vi "OAT Order Power Spectrum (N Channels).vi"(0 "even-angle signals":cluster{"r0":dbl, "dr":dbl, "Y":dbl[]}[](array[cluster]) {"r0" format="%.2p"; "dr" format="%.2p"; "Y" format="%.2f"}, 1 "dB on? (T)":bool=TRUE, 5 "even-angle channel info":T8[](array[typedef]) {"channel info"."pregain" format="%.2f"; "channel info"."weighting filter" items=["Linear", "A-weighting", "B-weighting", "C-weighting", "ITU-R 468-4", "Dolby", "CCITT", "C-message", "Wb", "Wc", "Wd", "We", "Wf", "Wh", "Wj", "Wk", "Wm", "AES17 20 kHz lowpass", "AES17 40 kHz lowpass", "AES17 20 kHz highpass", "AES17 40 kHz highpass"]; "channel info"."dB reference" format="%^.1e"; "channel info"."engineering units" items=["custom..."=0, "V"=1, "A"=21, "C"=30, "pC"=31, "s"=32, "-"=29, "Pa"=2, "N"=20, "g"=3, "m/s^2"=4, "m/s"=5, "m"=6, "mm/s"=12, "mm"=13, "micron/s"=14, "micron"=15, "in/s^2"=7, "in/s"=8, "in"=9, "mil/s"=10, "mil"=11, "rad/s^2"=16, "rad/s"=17, "rad"=18, "deg/s^2"=26, "deg/s"=27, "deg"=28, "RPM"=22, "cycle/s^2"=23, "Hz"=24, "cycle"=25, "strain"=19]; "channel info"."sensor sensitivity" format="%#_5f"}, 7 "window":u32(ring)=1 items=["None"=0, "Hanning"=1, "Hamming"=2, "Blackman-Harris"=3, "Exact Blackman"=4, "Blackman"=5, "Flat Top"=6, "4 Term B-Harris"=7, "7 Term B-Harris"=8, "Low Sidelobe"=9, "Gaussian"=62], 9 "block size":i32=1024 min=2, 11 "error in (no error)":errorcluster, 12 "averaging parameters":T7={"averaging mode"=enum."No averaging", "weighting mode"=enum."Exponential", "number of averages"=10, "linear mode"=enum."One shot"} {"number of averages" min=1 step=1}, 13 "restart averaging? (F)":bool) -> (3 "new spectrum available?":bool, 4 "order power spectra":T10(array[cluster]) {"order 0" format="%.2p"; "delta order" format="%.2p"; "magnitude" format="%.2f"}, 6 "unit labels":string[](array[string]), 8 "averages completed":dbl, 10 "spectrum info":T1[](array[typedef]) {"x-axis units" items=["Time (s)"=0, "Frequency-CB (Hz)"=1, "Frequency-CPB (Hz)"=1248, "Frequency-Arbitrary (Hz)"=2357, "Quefrency (s)"=2, "Revolutions (rev)"=3, "Order"=4, "Speed (RPM)"=11, "Speed (rad/s)"=21, "Index"=65535]; "weighting filter" items=["Linear", "A-weighting", "B-weighting", "C-weighting", "ITU-R 468-4", "Dolby", "CCITT", "C-message", "Wb", "Wc", "Wd", "We", "Wf", "Wh", "Wj", "Wk", "Wm", "AES17 20 kHz lowpass", "AES17 40 kHz lowpass", "AES17 20 kHz highpass", "AES17 40 kHz highpass"]; "dB reference [EU]" format="%.2f"; "engineering units" items=["custom..."=0, "V"=1, "A"=21, "C"=30, "pC"=31, "s"=32, "-"=29, "Pa"=2, "N"=20, "g"=3, "m/s^2"=4, "m/s"=5, "m"=6, "mm/s"=12, "mm"=13, "micron/s"=14, "micron"=15, "in/s^2"=7, "in/s"=8, "in"=9, "mil/s"=10, "mil"=11, "rad/s^2"=16, "rad/s"=17, "rad"=18, "deg/s^2"=26, "deg/s"=27, "deg"=28, "RPM"=22, "cycle/s^2"=23, "Hz"=24, "cycle"=25, "strain"=19]; "spectral info"."window" items=["None "=0, "Hanning"=1, "Hamming"=2, "Blackman-Harris"=3, "Exact Blackman"=4, "Blackman"=5, "Flat Top"=6, "4 Term B-Harris "=7, "7 Term B-Harris"=8, "Low Sidelobe"=9, "Force - Exponential"=10, "Gaussian"=62]}, 14 "averaging done?":bool, 15 "error out":errorcluster)   [LabVIEW 2017, in "SoundVib_OrderTracking.lvlib"]
doc: "Computes the order power spectrum of an even-angle signal. Wire data to the <B>even-angle signal</B> input to determine the polymorphic instance to use or manually select the instance."
uses:
  <vilib>/addons/Sound and Vibration/Order Analysis/Resample Order Tracking/SoundVib_OrderTracking.lvlib
  <vilib>/addons/_NISVFA/_Shared subVIs/Controls/svc_Resampled Channel Info.ctl
  <vilib>/addons/_NISVFA/_Shared subVIs/Controls/svc_Channel Info.ctl
  <vilib>/addons/_NISVFA/_Shared subVIs/Controls/svc_Engineering Units Text Ring.ctl
  <vilib>/addons/_NISVFA/_Shared subVIs/Controls/svc_Weighting Filter Text Ring.ctl
  <vilib>/addons/_NISVFA/_Shared subVIs/Controls/svc_Spectrum Info.ctl
  <vilib>/addons/_NISVFA/_Shared subVIs/Controls/svc_X-Axis Units.ctl
  <vilib>/addons/_NISVFA/_Shared subVIs/Controls/svc_Spectrum Type.ctl
  <vilib>/addons/_NISVFA/_Shared subVIs/Controls/svc_Complimentary Spectrum Units.ctl
  <vilib>/addons/Sound and Vibration/Order Analysis/Resample Order Tracking/SoundVib_Resampling.lvlib
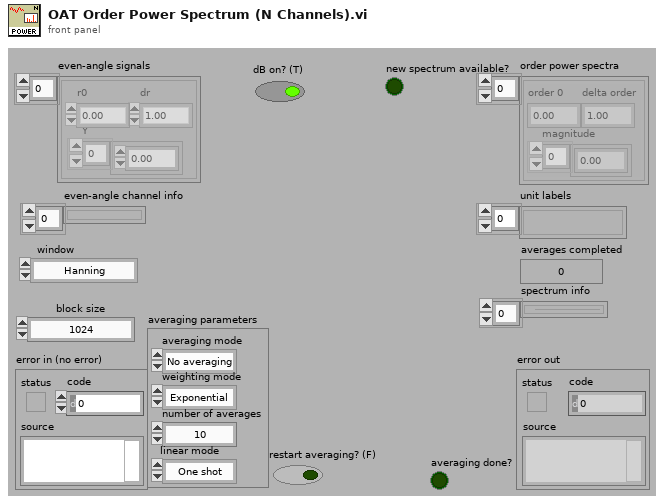
[diagram p1: front panel]
types:
  T1 = typedef "svc_Spectrum Info.ctl" = cluster{"channel name":string, "description":string, "x-axis units":T2, "spectral info":cluster{"spectrum type":T3, "linear/dB":enum16{"linear", "dB"}, "window":u16, "window size":i32, "FFT size":i32}, "engineering units":T4, "custom label":string, "dB reference [EU]":dbl, "peak units":enum16{"rms", "peak", "peak-peak"}, "weighting filter":T5, "spectral density?":bool, "unit label":string, "spectrum skewed?":bool, "complimentary spectrum units":T6}
  T2 = typedef "svc_X-Axis Units.ctl" = u16
  T3 = typedef "svc_Spectrum Type.ctl" = enum16{"FFT Spectrum [complex]", "Amplitude [Magnitude]", "Power [Magnitude^2]", "Cross Spectrum [complex]", "Frequency Response [Complex]"}
  T4 = typedef "svc_Engineering Units Text Ring.ctl" = u16
  T5 = typedef "svc_Weighting Filter Text Ring.ctl" = u16
  T6 = typedef "svc_Complimentary Spectrum Units.ctl" = enum16{"none", "radians", "degrees", "cycles", "imaginary"}
  T7 = cluster{"averaging mode":enum16{"No averaging", "Vector averaging", "RMS averaging", "Peak hold"}, "weighting mode":enum16{"Linear", "Exponential"}, "number of averages":u32, "linear mode":enum16{"One shot", "Auto restart"}}
  T8 = typedef "svc_Resampled Channel Info.ctl" = cluster{"channel name":string, "description":string, " channel info":T9}
  T9 = typedef "svc_Channel Info.ctl" = cluster{"sensor sensitivity":dbl, "engineering units":T4, "dB reference":dbl, "custom label":string, "weighting filter":T5, "pregain":dbl}
  T10 = cluster{"order 0":dbl, "delta order":dbl, "magnitude":dbl[]}[]
  T11 = cluster{"ignore dt":bool, "ignore t0 continuity":bool, "ignore array length":bool, "ignore channel info":bool, "ignore channel name":bool}
  T12 = cluster{"ignore dt's equal":bool, "ignore array lengths equal":bool, "ignore # channels":bool}
  T13 = cluster{"r0":dbl, "dr":dbl, "even angle signal":dbl[]}[]
  T14 = enum16{"Restart processing", "Continue processing", "Skip processing"}
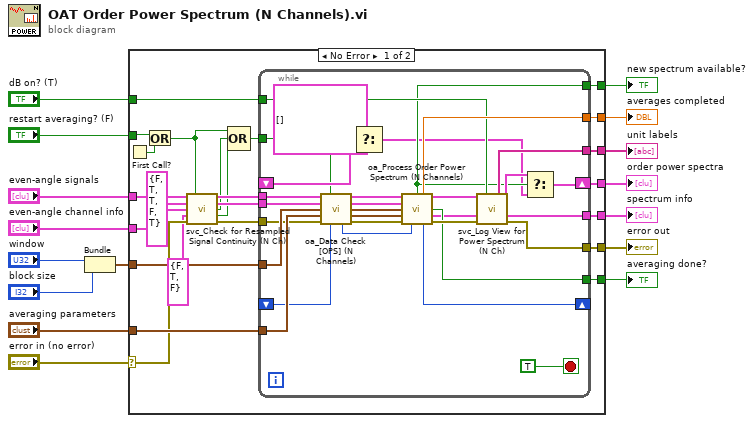
[diagram p0: block diagram]
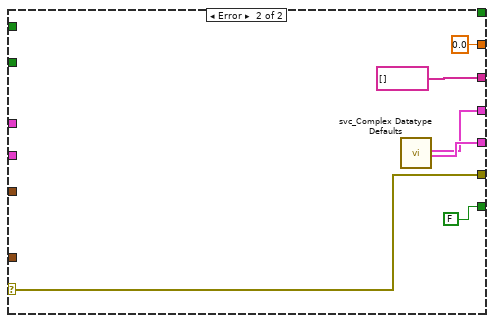
[diagram p2: hidden frame]
diagram:
  n1 = Bundle("window"="window", "block size"="block size") -> (w10:cluster{"window":u32, "block size":i32})  [unwired: 1 in]
  n2 = case shown="No Error" "error in (no error)" {
    selector: "error in (no error)" -> [w24 w76]
    tunnel: "even-angle signals" -> [w28 _]
    tunnel: "averaging parameters" -> [w40 _]
    tunnel: "restart averaging? (F)" -> [w29 _]
    tunnel: "even-angle channel info" -> [w26 _]
    tunnel: "dB on? (T)" -> [w39 _]
    tunnel: [w38 w76] -> w7
    tunnel: [w37 w73] -> w2
    tunnel: [w36 w72] -> w4
    tunnel: [w35 string[] []] -> w3
    tunnel: [w34 0.0 ("averages completed")] -> w5
    tunnel: [w33 FALSE ("averaging done")] -> w6
    tunnel: w10 -> [w32 _]
    tunnel: [w31 _] -> w1
    frame No Error {
      n3 = First Call?() -> (First Call?: T/F=w30:bool)
      n4 = Or(x=w29, y=w30) -> (x .or. y?=w21:bool)
      n5 = call <vilib>:"svc_Check for Resampled Signal Continuity (N Ch).vi"("even angle signals"=w28, "restart averaging (F)"=w21, "even angle channel info"=w26, "parameter controls"=T11 {"ignore dt"=FALSE, "ignore t0 continuity"=TRUE, "ignore array length"=TRUE, "ignore channel info"=FALSE, "ignore channel name"=TRUE}, "multichannel parameter controls"=T12 {"ignore dt's equal"=FALSE, "ignore array lengths equal"=TRUE, "ignore # channels"=FALSE}, "error in (no error)"=w24) -> ("dup even angle signals"=w27:T13, "dup even angle channel info"=w25:T8[], "waveform parameter changed"=w20:bool, "multichannel parameter changed"=w19:bool, "error out"=w23:errorcluster)  [unwired: 3 in, 2 out]
      n6 = Compound Arithmetic op=OR(w21, w20, w19) -> (w22:bool)
      n7 = while {
        tunnel: w27 -> [w70]
        tunnel: w40 -> [w69]
        tunnel: w25 -> [w53]
        tunnel: w39 -> [w49]
        tunnel: [w62] -> w38
        tunnel: [w61] -> w37
        tunnel: [w60] -> w35
        tunnel: [w59] -> w34
        tunnel: [w58] -> w33
        shift-right: [w55] -> _
        shift-left: _ -> [w56]
        tunnel: w32 -> [w54]
        tunnel: [w44] -> w31
        shift-right: [w45] -> w36
        shift-left: _ -> [w48]
        tunnel: w23 -> [w42]
        tunnel: w22 -> [w41]
        stop <- TRUE stop-if-true
        n8 = call <vilib>:"oa_Data Check [OPS] (N Channels).vi"("resampled signals"=w70, "restart averaging (F)"=w41, "channel info"=w53, "spectrum settings"=w54, "averaging parameters"=w69, "error in (no error)"=w42, "processing control in"=w56) -> ("dup resampled signals"=w64:cluster{"r0":dbl, "dr":dbl, "Y":dbl[]}[], "dup channel info"=w52:T8[], "dup spectrum settings"=w65:cluster{"window type":u32, "block size":i32}, "dup averaging parameters"=w66:T7, "processing control out"=w68:T14, "error out"=w67:errorcluster)  [unwired: 3 in]
        n9 = Select(t=cluster{"f0":dbl, "df":dbl, "spectrum":dbl[]}[] [], s=w41, f=w48) -> (s? t:f=w43:cluster{"f0":dbl, "df":dbl, "spectrum":dbl[]}[])
        n10 = call <vilib>:"oa_Process Order Power Spectrum (N Channels).vi"("even angle signals"=w64, "channel info"=w52, "spectrum settings"=w65, "averaging parameters"=w66, "error in"=w67, "processing control in"=w68) -> ("new spectrum available?"=w44:bool, "averages completed"=w59:dbl, "order power spectrum"=w51:T10, "averaging done"=w58:bool, "spectrum info"=w50:T1[], "processing control out"=w55:T14, "error out"=w63:errorcluster)  [unwired: 3 in]
        n11 = call <vilib>:"svc_Log View for Power Spectrum (N Ch).vi"("Power Spectra [EU^2 rms]"=w51, "dB On (F)"=w49, "spectra info in"=w50, "error in (no error)"=w63) -> ("unit label(s)"=w60:string[], "Power Spectra [EU^2 rms]"=w46:cluster{"f0":dbl, "df":dbl, "spectrum":dbl[]}[], "spectra info out"=w61:T1[], "error out"=w62:errorcluster)  [unwired: 8 in]
        n12 = Select(t=w46, s=w44, f=w43) -> (s? t:f=w45:cluster{"f0":dbl, "df":dbl, "spectrum":dbl[]}[])
      }
    }
    frame Error {
      n13 = call <vilib>:"svc_Complex Datatype Defaults.vi"() -> ("empty array of spectra"=w72:cluster{"f0":dbl, "df":dbl, "magnitude":dbl[]}[], "empty array of spectrum info"=w73:T1[])  [unwired: 11 in, 7 out]
    }
  }
  "error out" <- w7
  "order power spectra" <- w4
  "unit labels" <- w3
  "averaging done?" <- w6
  "averages completed" <- w5
  "spectrum info" <- w2
  "new spectrum available?" <- w1
